vi "拷贝创建文件夹.vi"(0 "产品型号路径":path, 5 "产品型号":string="potteryTemplete", 7 "新型号":string="potteryTemplete", 11 "error in (no error)":errorcluster caption="错误输入（无错误）") -> (15 "error out":errorcluster caption="错误输出")   [LabVIEW 2017]
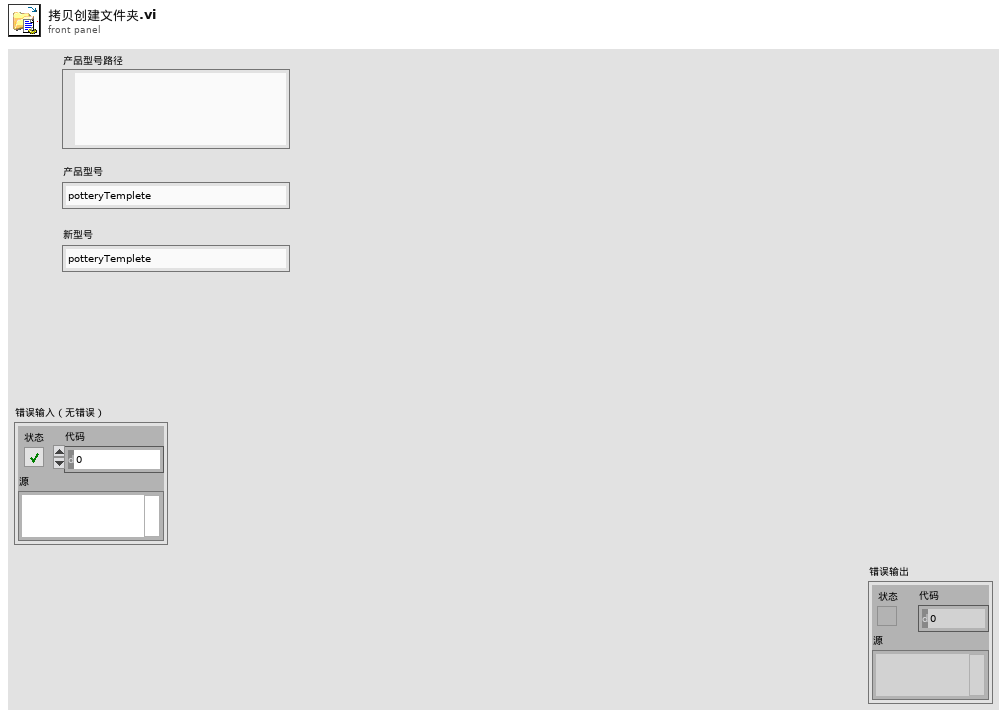
[diagram p1: front panel]
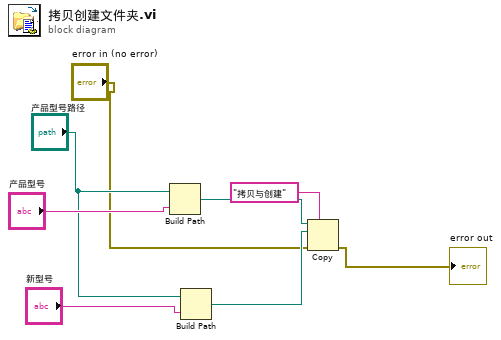
[diagram p0: block diagram]
diagram:
  n1 = Build Path(base path="产品型号路径", name or relative path="产品型号") -> (appended path=w6:path)
  n2 = Build Path(base path="产品型号路径", name or relative path="新型号") -> (appended path=w4:path)
  n3 = Copy(7:"拷贝与创建" ("对话框窗口（选择或输入文件路径）"), 8:"error in (no error)", 10:w4, 11:w6) -> (0:→"error out":errorcluster)  [unwired: 1 in, 2 out]
